vi "Get Events.vi"(11 "Create Test Node View in":refnum<class "Edit Test Node View.lvclass">) -> (2 "Events":T1, 3 "Create Test Node View out":refnum<class "Edit Test Node View.lvclass">)   [LabVIEW 2013, in "Edit Test Node View.lvlib" / "Edit Test Node View.lvclass"]
uses:
  Edit Test Node View.lvclass
  Typedef/Events.ctl
  Edit Test Node View.lvclass/Edit Test Node View.ctl
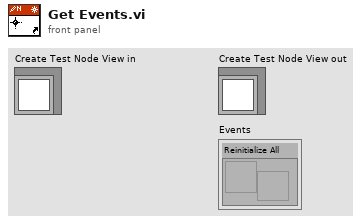
[diagram p1: front panel]
types:
  T1 = typedef "Edit Test Node View.lvlib/Edit Test Node View.lvclass/Events.ctl" = cluster{"Reinitialize All":refnum<user-event>}
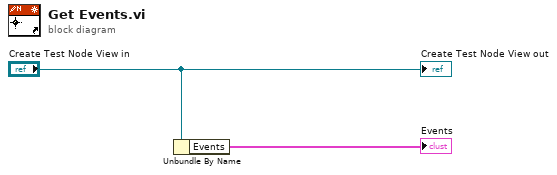
[diagram p0: block diagram]
diagram:
  n1 = Unbundle By Name("Create Test Node View in") -> ("Events"=→"Events":T1)
  "Create Test Node View out" <- "Create Test Node View in"
